vi "Expansion Dequeue.vi"(8 "error in (no error)":errorcluster, 11 "Queue in":refnum<queue>) -> (0 "error out":errorcluster, 1 "Data":variant, 2 "State":T1, 3 "Queue out":refnum<queue>)   [LabVIEW 2017, in "Expansion.lvclass"]
uses:
  Expansion.lvclass
  Type Defs/Expansion State.ctl
  Expansion.lvclass/Expansion.ctl
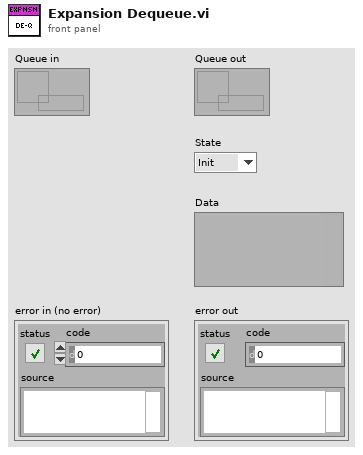
[diagram p1: front panel]
types:
  T1 = typedef "Expansion.lvclass/Expansion State.ctl" = enum16{"Init", "Update", "Go", "Move from Load to Heating", "Stop Motor", "Operate Cylinders", "Wait and Monitor", "Move from Heating to Unload", "Unload", "Move from Unload to Heating", "Move from Heating to Load", "Complete Process", "Stop", "Idle", "Error", "Shutdown"}
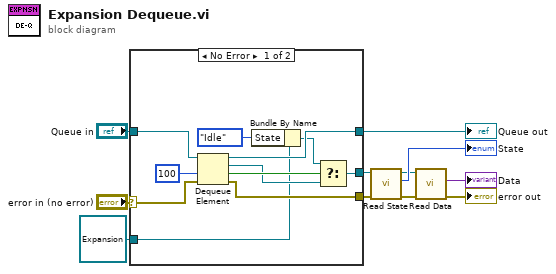
[diagram p0: block diagram]
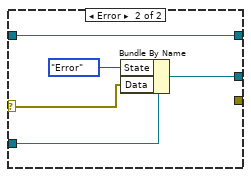
[diagram p2: hidden frame]
diagram:
  n1 = case shown="No Error" "error in (no error)" {
    selector: "error in (no error)" -> [w21 w24]
    tunnel: "Queue in" -> [w22 w27]
    tunnel: [w15 w26] -> w7
    tunnel: [w20 w27] -> w10
    tunnel: [w19 _] -> w6
    tunnel: refnum<class "Expansion.lvclass"> refnum ("Expansion.lvclass") -> [w12 w23]
    frame No Error {
      n2 = Dequeue Element(queue=w22, timeout in ms (-1)=100, error in (no error)=w21) -> (queue out=w20:refnum<queue>, element=w16:refnum<class "Expansion.lvclass">, timed out?=w17:bool, error out=w19:errorcluster)
      n3 = Bundle By Name(cluster=w12, "State"=Expansion_State."Idle") -> (w14:refnum<class "Expansion.lvclass">)
      n4 = Select(t=w14, s=w17, f=w16) -> (s? t:f=w15:refnum<class "Expansion.lvclass">)
    }
    frame Error {
      n5 = Bundle By Name(cluster=w23, "State"=Expansion_State."Error", "Data"=w24) -> (w26:refnum<class "Expansion.lvclass">)
    }
  }
  "Queue out" <- w10
  n6 = call "Read State.vi"("error in (no error)"=w6, "Expansion in"=w7) -> ("error out"=w3:errorcluster, "State"=→"State":T1, "Expansion out"=w5:refnum<class "Expansion.lvclass">)  [unwired: 7 in]
  n7 = call "Read Data.vi"("error in (no error)"=w3, "Expansion in"=w5) -> ("error out"=→"error out":errorcluster, "Data"=→"Data":variant)  [unwired: 7 in, 1 out]
